vi "Apply One Port Correction Factors - e10e01.vi"(0 "Raw Sxx Data":cdb[](array[numeric]), 7 "One Port Correction Factors":cdb[][](array[numeric]), 11 "Error In":errorcluster) -> (4 "Corrected Sxx Data":cdb[](array[numeric]), 15 "Error Out":errorcluster)   [LabVIEW 2013]
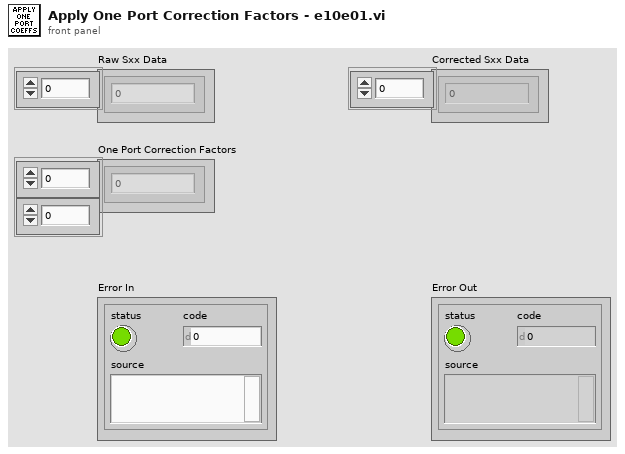
[diagram p1: front panel]
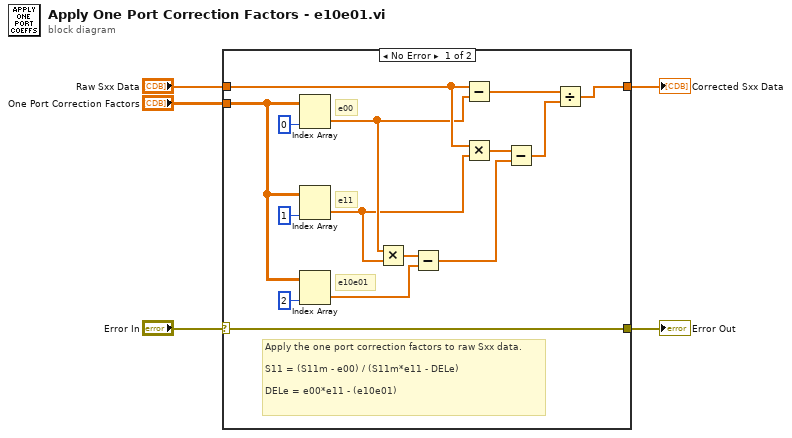
[diagram p0: block diagram]
diagram:
  n1 = case shown="No Error" "Error In" {
    selector: "Error In" -> [w11 w21]
    tunnel: "Raw Sxx Data" -> [w18 w22]
    tunnel: "One Port Correction Factors" -> [w16 _]
    tunnel: [w12 w22] -> w4
    tunnel: [w11 w21] -> w2
    frame No Error {
      # "e10e01"
      # "e11"
      # "e00"
      # "Apply the one port correction factors to raw Sxx data.\n\nS11 = (S11m - e00) / (S11m*e11 - DELe)\n\nDELe = e00*e11 - (e10e01)"
      n2 = Index Array(array=w16, index (col)=0 ("disabled index (col)")) -> (element=w10:cdb[])  [unwired: 1 in]
      n3 = Index Array(array=w16, index (col)=1 ("disabled index (col)")) -> (element=w9:cdb[])  [unwired: 1 in]
      n4 = Index Array(array=w16, index (col)=2 ("disabled index (col)")) -> (element=w7:cdb[])  [unwired: 1 in]
      n5 = Multiply(x=w10, y=w9) -> (x*y=w8:cdb[])
      n6 = Subtract(x=w8, y=w7) -> (x-y=w6:cdb[])
      n7 = Subtract(x=w18, y=w10) -> (x-y=w20:cdb[])
      n8 = Multiply(x=w18, y=w9) -> (x*y=w17:cdb[])
      n9 = Subtract(x=w17, y=w6) -> (x-y=w19:cdb[])
      n10 = Divide(x=w20, y=w19) -> (x/y=w12:cdb[])
    }
    frame Error {
    }
  }
  "Corrected Sxx Data" <- w4
  "Error Out" <- w2
